vi "LinearConvertion.vi"(0 "Input":dbl, 1 "Factors":T1={"a"=1.0, "b"=0.0}) -> (2 "Output":dbl)   [LabVIEW 2012]
uses:
  LinearFactors.ctl
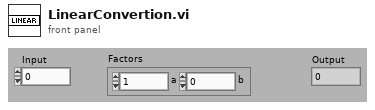
[diagram p1: front panel]
types:
  T1 = typedef "LinearFactors.ctl" = cluster{"a":dbl, "b":dbl}
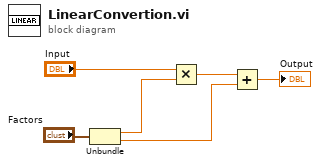
[diagram p0: block diagram]
diagram:
  n1 = Unbundle("Factors") -> ("a"=w4:dbl, "b"=w2:dbl)
  n2 = Multiply(x="Input", y=w4) -> (x*y=w3:dbl)
  n3 = Add(x=w3, y=w2) -> (x+y=→"Output":dbl)
